vi "aquire_image.vi"(0 "IMAQ Session In":refnum<k11>, 2 "Buffer to extract":i32, 7 "Imaging Variables In":T1, 11 "error in (no error)":errorcluster, 12 "Img Q Data In":T2) -> (4 "IMAQ Session Out":refnum<k11>, 8 "Imaging Variables Out":T1, 14 "Img Q Data Out":T2, 15 "error out":errorcluster)   [LabVIEW 2023]
uses:
  <vilib>/vision/Image Controls.llb/IMAQ Image.ctl
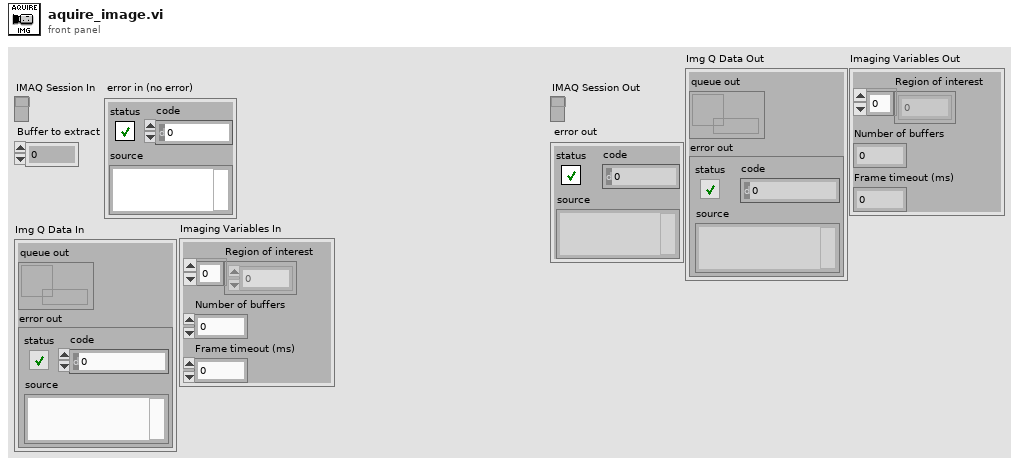
[diagram p1: front panel]
types:
  T1 = cluster{"Region of interest":i32[], "Number of buffers":u32, "Frame timeout (ms)":u32}
  T2 = cluster{"queue out":refnum<queue>, "error out":errorcluster}
  T3 = typedef "IMAQ Image.ctl" = refnum<image>
  T4 = cluster{"Image Out":T3, "Image Data":cluster{"Actual Width":u32, "Actual Height":u32, "Buffer Number":i32}, "Imaging Variables In":cluster{"Region of interest":i32[], "Number of buffers":u32, "Frame timeout (ms)":u32}}
  T5 = cluster{"Actual Width":u32, "Actual Height":u32, "Buffer Number":i32}
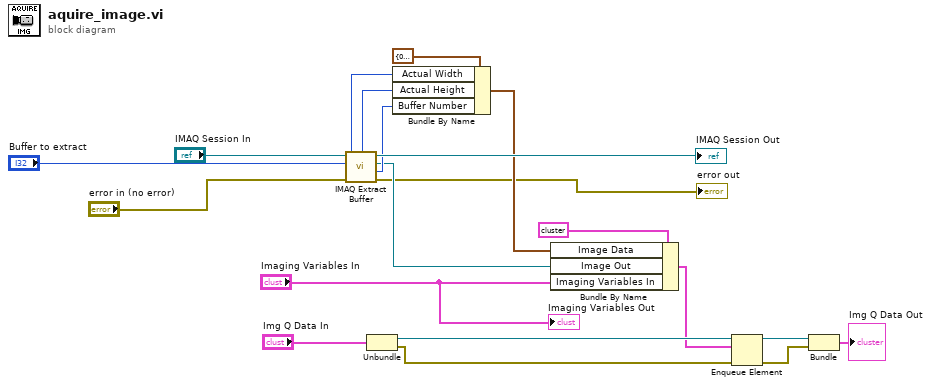
[diagram p0: block diagram]
diagram:
  n1 = call <vilib>:"IMAQ Extract Buffer.vi"("error in (no error)"="error in (no error)", "Buffer to extract"="Buffer to extract", "IMAQ Session In"="IMAQ Session In") -> ("error out"=→"error out":errorcluster, "Buffer Number"=w13:i32, "Image Out"=w11:T3, "IMAQ Session Out"=→"IMAQ Session Out":refnum<k11>, "Actual Height"=w14:u32, "Actual Width"=w15:u32)  [unwired: 3 in]
  n2 = Unbundle("Img Q Data In") -> ("queue out"=w8:refnum<queue>, "error out"=w4:errorcluster)
  n3 = Bundle By Name(cluster=T5 {"Actual Width"=0, "Actual Height"=0, "Buffer Number"=0}, "Actual Width"=w15, "Actual Height"=w14, "Buffer Number"=w13) -> (w12:T5)
  n4 = Bundle By Name(cluster=T4 {"Image Out"=refnum, "Image Data"={"Actual Width"=0, "Actual Height"=0, "Buffer Number"=0}, "Imaging Variables In"={"Region of interest"=[], "Number of buffers"=0, "Frame timeout (ms)"=0}} ("output cluster"), "Image Data"=w12, "Image Out"=w11, "Imaging Variables In"="Imaging Variables In") -> (w5:T4)
  n5 = Enqueue Element(queue=w8, element=w5, error in (no error)=w4) -> (queue out=w3:refnum<queue>, error out=w2:errorcluster)  [unwired: 1 in, 1 out]
  n6 = Bundle("queue out"=w3, "error out"=w2) -> (→"Img Q Data Out":T2)  [unwired: 1 in]
  "Imaging Variables Out" <- "Imaging Variables In"
